vi "Test Serialize.vi"() -> ()   [LabVIEW 2019, in "Instrument.Lockin.lvlib" / "Instrument.DAQ.lvclass"]
uses:
  Instrument.DAQ.lvclass
  Typedefs/PublicEvents--DAQ.getWaveforms.ctl
  Typedefs/REF.Channel--Cluster--Array.ctl
  Typedefs/REF.Channel--Cluster.ctl
  8d9fda7c-1aab-4e7d-9f20-08de648b59a2.vi
  396a608c-179a-4c97-aca9-f16702cc7d77.vi
  <vilib>/JDP Science/JSONtext/Variant to JSON Text.vi
  <vilib>/JDP Science/JSONtext/JSON text to Variant.vi
  <vilib>/JDP Science/JSONtext/LVClass Serializer/JSONtext LVClass Serializer.lvclass
  <vilib>/measure/NI_MABase.lvlib
panel:
  out "data 2":T1 {"Roll-Off" min=1 max=4; "TC" min=1e-06 max=100.0 format="%#_3p"; "Phase" format="%#_3p"; "Frequency" min=1e-06 max=102400.0 format="%#_6p"; "Channel" min=1}
  out "data":T3
  out "Flatten":dbl
  out "Unflatten":dbl
  out "JSON unserialize":dbl
  out "JSON serialize":dbl
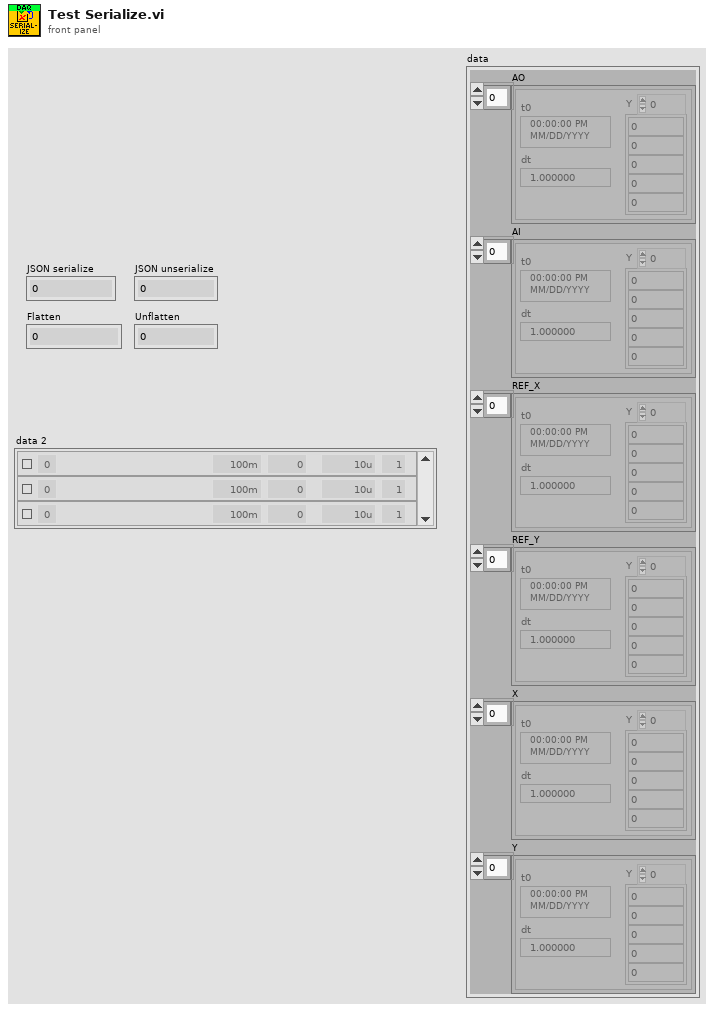
[diagram p1: front panel]
types:
  T1 = typedef "Instrument.Lockin.lvlib/Instrument.DAQ.lvclass/REF.Channel--Cluster--Array.ctl" = T2[]
  T2 = typedef "Instrument.Lockin.lvlib/Instrument.DAQ.lvclass/REF.Channel--Cluster.ctl" = cluster{"Enable?":bool, "Channel":i32, "Frequency":dbl, "Phase":dbl, "TC":dbl, "Roll-Off":i32}
  T3 = typedef "Instrument.Lockin.lvlib/Instrument.DAQ.lvclass/PublicEvents--DAQ.getWaveforms.ctl" = cluster{"AO":waveform(dbl)[], "AI":waveform(dbl)[], "REF_X":waveform(dbl)[], "REF_Y":waveform(dbl)[], "X":waveform(dbl)[], "Y":waveform(dbl)[]}
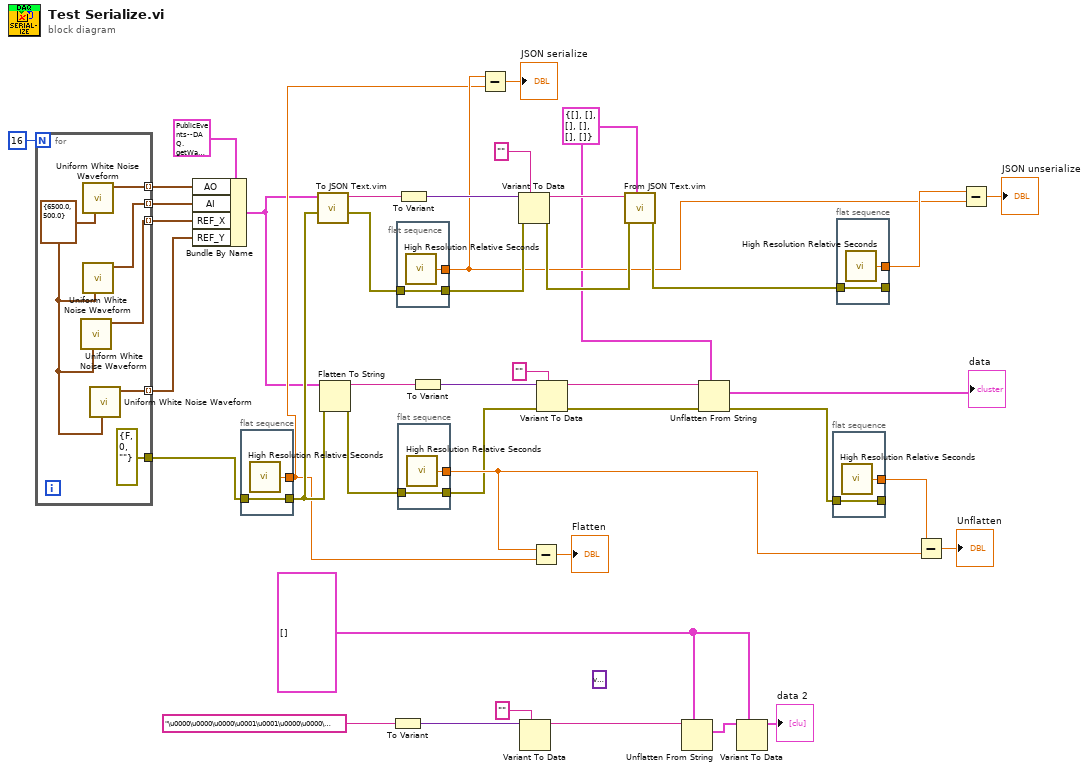
[diagram p0: block diagram]
diagram:
  (unwired) variant
  w1 = T1 [] ("REF Channels")
  w14 = T3 {"AO"=[], "AI"=[], "REF_X"=[], "REF_Y"=[], "X"=[], "Y"=[]} ("Waveforms")
  n1 = for {
    N: 16 -> [_]
    tunnel: [w49] -> w31 mode=indexing
    tunnel: [w48] -> w30 mode=indexing
    tunnel: [w47] -> w29 mode=indexing
    tunnel: [w46] -> w15 mode=indexing
    tunnel: [errorcluster {"status"=FALSE, "code"=0, "source"=""} ("error out")] -> w27
    w45 = cluster{"Fs":dbl, "#s":dbl} {"Fs"=6500.0, "#s"=500.0} ("sampling info")
    n2 = call <vilib>:"Uniform White Noise Waveform.vi"("sampling info"=w45) -> ("signal out"=w47:waveform(dbl))  [unwired: 9 in, 1 out]
    n3 = call <vilib>:"Uniform White Noise Waveform.vi"("sampling info"=w45) -> ("signal out"=w49:waveform(dbl))  [unwired: 9 in, 1 out]
    n4 = call <vilib>:"Uniform White Noise Waveform.vi"("sampling info"=w45) -> ("signal out"=w48:waveform(dbl))  [unwired: 9 in, 1 out]
    n5 = call <vilib>:"Uniform White Noise Waveform.vi"("sampling info"=w45) -> ("signal out"=w46:waveform(dbl))  [unwired: 9 in, 1 out]
  }
  n6 = Bundle By Name(cluster=T3 {"AO"=[{"t0"=timestamp(0 s since 1904-01-01), "dt"=1.0, "Y"=[0.0, 1.0]}], "AI"=[{"t0"=timestamp(0 s since 1904-01-01), "dt"=1.0, "Y"=[0.0, 1.0]}], "REF_X"=[], "REF_Y"=[], "X"=[], "Y"=[]} ("Waveforms"), "AO"=w31, "AI"=w30, "REF_X"=w29, "REF_Y"=w15) -> (w16:T3)
  n7 = flat-sequence {
    tunnel: [w51] -> w37
    tunnel: w27 -> [w51]
    tunnel: [w50] -> w18
    frame #0 {
      n8 = call <vilib>:"High Resolution Relative Seconds.vi"() -> ("relative seconds"=w50:dbl)
    }
  }
  n9 = call "To JSON Text.vim"("error in (no error)"=w37, "Anything"=w16) -> ("error out"=w36:errorcluster, "<JSON>"=w40:string)  [unwired: 8 in]
  n10 = Flatten To String(anything=w16, error in (no error)=w37) -> (data string=w13:string, error out=w38:errorcluster)  [unwired: 2 in, 1 out]
  n11 = To Variant(anything="\u0000\u0000\u0000\u0001\u0001\u0000\u0000\u0000\u0001@*\u0000\u0000\u0000\u0000\u0000\u0000\u0000\u0000\u0000\u0000\u0000\u0000\u0000\u0000?¹™™™™™š\u0000\u0000\u0000\u0002" ("Data")) -> (Variant=w3:variant)
  n12 = flat-sequence {
    tunnel: [w53] -> w35
    tunnel: w36 -> [w53]
    tunnel: [w52] -> w23
    frame #0 {
      n13 = call <vilib>:"High Resolution Relative Seconds.vi"() -> ("relative seconds"=w52:dbl)
    }
  }
  n14 = flat-sequence {
    tunnel: [w55] -> w9
    tunnel: w38 -> [w55]
    tunnel: [w54] -> w19
    frame #0 {
      n15 = call <vilib>:"High Resolution Relative Seconds.vi"() -> ("relative seconds"=w54:dbl)
    }
  }
  n16 = To Variant(anything=w40) -> (Variant=w41:variant)
  n17 = To Variant(anything=w13) -> (Variant=w11:variant)
  n18 = Subtract(x=w23, y=w18) -> (x-y=→"JSON serialize":dbl)
  n19 = Variant To Data(error in=w35, type="", Variant=w41) -> (data=w42:string, error out=w34:errorcluster)
  n20 = Variant To Data(type="", Variant=w3) -> (data=w7:string)  [unwired: 1 in, 1 out]
  n21 = Subtract(x=w19, y=w18) -> (x-y=→"Flatten":dbl)
  n22 = Variant To Data(error in=w9, type="", Variant=w11) -> (data=w10:string, error out=w8:errorcluster)
  n23 = call "From JSON Text.vim"("Data Type and Default Value"=w14, "error in (no error)"=w34, "JSON"=w42) -> ("error out"=w33:errorcluster)  [unwired: 7 in, 1 out]
  n24 = Unflatten From String(type=w1, binary string=w7) -> (value=w5:T1)  [unwired: 3 in, 2 out]
  n25 = Unflatten From String(type=w14, binary string=w10, error in (no error)=w8) -> (value=→"data":T3, error out=w39:errorcluster)  [unwired: 2 in, 1 out]
  n26 = Variant To Data(type=w1, Variant=w5) -> (data=→"data 2":T1)  [unwired: 1 in, 1 out]
  n27 = flat-sequence {
    tunnel: [w57] -> _
    tunnel: w39 -> [w57]
    tunnel: [w56] -> w20
    frame #0 {
      n28 = call <vilib>:"High Resolution Relative Seconds.vi"() -> ("relative seconds"=w56:dbl)
    }
  }
  n29 = flat-sequence {
    tunnel: [w59] -> _
    tunnel: w33 -> [w59]
    tunnel: [w58] -> w24
    frame #0 {
      n30 = call <vilib>:"High Resolution Relative Seconds.vi"() -> ("relative seconds"=w58:dbl)
    }
  }
  n31 = Subtract(x=w20, y=w19) -> (x-y=→"Unflatten":dbl)
  n32 = Subtract(x=w24, y=w23) -> (x-y=→"JSON unserialize":dbl)
